vi "ModulateVBatOut SetControl.vi"(0 "DeviceReference":T1, 1 "Output":dbl, 7 "error in":errorcluster, 18 "Update Frequency (Hz)":dbl=100.0) -> (20 "DeviceReference Out":T1, 27 "error out":errorcluster)   [LabVIEW 2025]
doc: "Modulates the CANdle VBat output to the specified duty cycle. This can be used to control a single-color LED strip.\nNote that ${cfg}CANdleFeaturesConfigs$:VBatOutputMode must be set to $sVBatOutputModeValue$:Modulated."
uses:
  <vilib>/Rock Robotics/WPI/ThirdParty/Phoenix6/DeviceReference.ctl
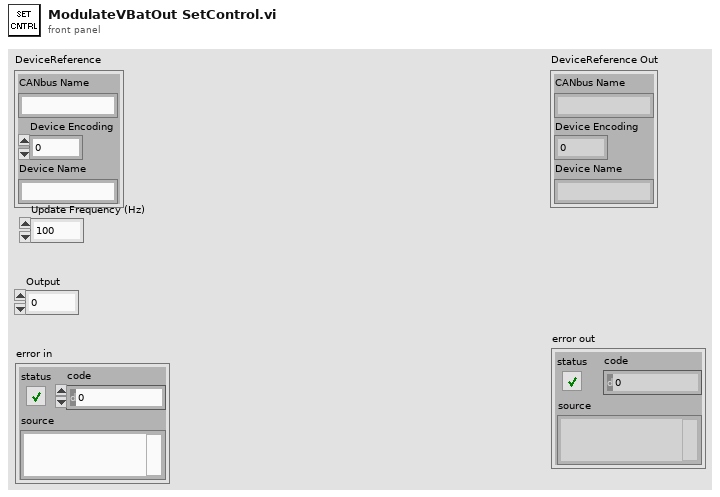
[diagram p1: front panel]
types:
  T1 = typedef "DeviceReference.ctl" = cluster{"CANbus Name":string, "Device Encoding":u32, "Device Name":string}
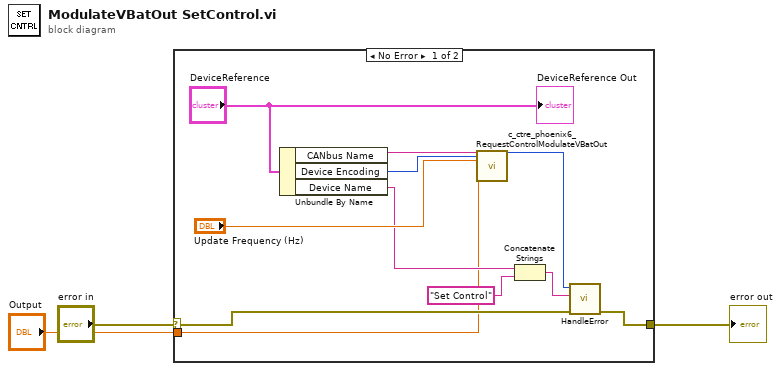
[diagram p0: block diagram]
diagram:
  n1 = case shown="No Error" "error in" {
    selector: "error in" -> [w9 w15]
    tunnel: [w8 w15] -> w2
    tunnel: "Output" -> [w4 _]
    frame No Error {
      n2 = Unbundle By Name("DeviceReference") -> ("CANbus Name"=w13:string, "Device Encoding"=w12:u32, "Device Name"=w7:string)
      n3 = call <vilib>:"c_ctre_phoenix6_RequestControlModulateVBatOut.vi"("String 2"=w13, "Numeric 2"=w12, "Numeric 3"="Update Frequency (Hz)", "Numeric 4"=w4) -> ("Numeric"=w10:i32)  [unwired: 22 in, 1 out]
      n4 = Concatenate Strings(w7, "Set Control" ("origin")) -> (w5:string)
      n5 = call <vilib>:"HandleError.vi"("error in"=w9, "origin"=w5, "Status"=w10) -> ("error out"=w8:errorcluster)  [unwired: 8 in]
      "DeviceReference Out" <- "DeviceReference"
    }
    frame Error {
    }
  }
  "error out" <- w2
